vi "MPB comm protocol.vi"(8 "error in":errorcluster) -> (0 "error out":errorcluster, 2 "value":T1={"MPB IP Address"="192.168.1.9", "MPB VLAN"="1", "MPB Port"="11111", "PCP IP Address"="192.168.1.123", "PC VLAN"="1", "PC Port"="11112"})   [LabVIEW 2020]
uses:
  controls/comm protocol auto ethernet.ctl
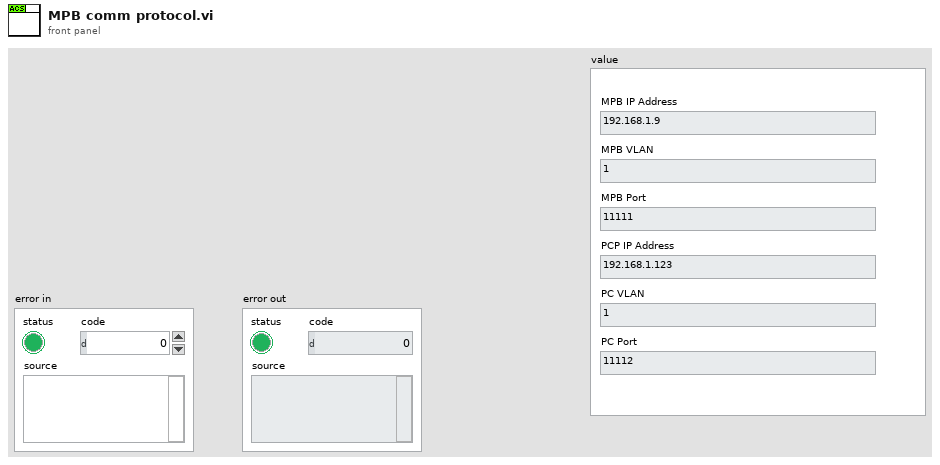
[diagram p1: front panel]
types:
  T1 = typedef "comm protocol auto ethernet.ctl" = cluster{"MPB IP Address":string, "MPB VLAN":string, "MPB Port":string, "PCP IP Address":string, "PC VLAN":string, "PC Port":string}
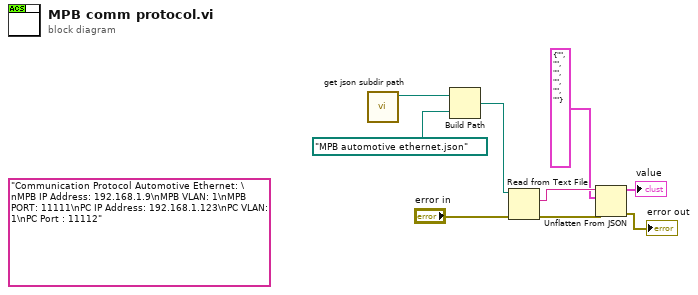
[diagram p0: block diagram]
diagram:
  (unwired) "Communication Protocol Automotive Ethernet: \nMPB IP Address: 192.168.1.9\nMPB VLAN: 1\nMPB PORT: 11111\nPC IP Address: 192.168.1.123\nPC VLAN: 1\nPC Port : 11112"
  n1 = call "get json subdir path.vi"() -> ("json path"=w9:path)  [unwired: 10 in, 1 out]
  n2 = Build Path(base path=w9, name or relative path=path "MPB automotive ethernet.json") -> (appended path=w7:path)
  n3 = Read from Text File(file (use dialog)=w7, error in="error in") -> (text=w6:string, error out=w3:errorcluster)  [unwired: 2 in, 2 out]
  n4 = Unflatten From JSON(JSON string=w6, type and defaults=T1 {"MPB IP Address"="", "MPB VLAN"="", "MPB Port"="", "PCP IP Address"="", "PC VLAN"="", "PC Port"=""} ("Communication Protocol Automotive Ethernet"), error in (no error)=w3) -> (value=→"value":T1, error out=→"error out":errorcluster)  [unwired: 4 in]
